vi "MCSPowerWriter.vi"(4 "ErrorIn":errorcluster, 5 "UDPResponse":string="\u0000\u0000PM\u001eš\n\u0000.¾\u0004\b\u0000\u0000\u00000\u0000\u0000\u00000\u0000\u0000\u00000\u0000\u0000\u00000\u0000\u0000\u00000«Î\u0004\b\u0000\u0000\u00000\u0000\u0000\u00000\u0000\u0000\u00000\u0000\u0000\u00000\u0000\u0000\u00000ÿÿÿÿ", 6 "MPDUnitID":T1=enum."MPD#04", 7 "PowerChannelMap":T2[](array[typedef])=[enum."WVOnline", enum."Unassigned", enum."Unassigned", enum."Unassigned", enum."Unassigned", enum."Unassigned", enum."WVOffline", enum."Unassigned", enum."Unassigned", enum."Unassigned", enum."Unassigned", enum."Unassigned"]) -> (0 "ErrorOut":errorcluster, 3 "ByteArray":u8[](array[numeric])=[64, 55, 34, 184, 91, 157, 14, 129, 0, 12, 0, 0, 0, 0, 0, 0, 1, 2, 3, 4, 5, 6, 0, 0, 80, 77, 30, 154, 10, 0, 46, 190, 4, 8, 0, 0, 0, 48, 0, 0, 0, 48, 0, 0, 0, 48, 0, 0, 0, 48, 0, 0, 0, 48, 171, 206, 4, 8, 0, 0, 0, 48, 0, 0, 0, 48, 0, 0, 0, 48, 0, 0, 0, 48, 0, 0, 0, 48, 255, 255, 255, 255, 13, 10])   [LabVIEW 2012]
uses:
  MCSPowerMap.ctl
  MPDUnitID.ctl
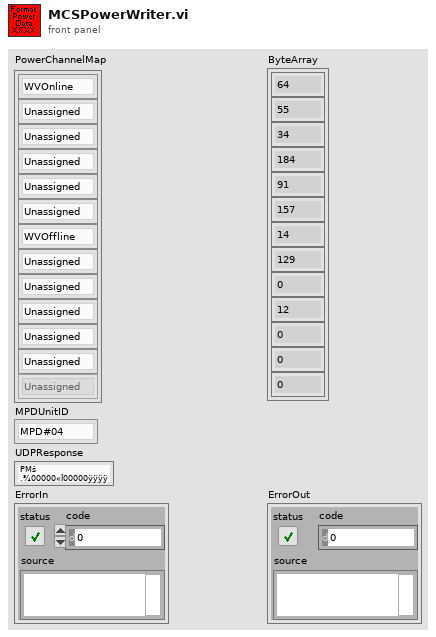
[diagram p1: front panel]
types:
  T1 = typedef "MPDUnitID.ctl" = enum8{"Unknown", "MPD#01", "MPD#02", "MPD#03", "MPD#04", "MPD#05"}
  T2 = typedef "MCSPowerMap.ctl" = enum8{"Unassigned", "Unknown", "WVOnline", "WVOffline", "O2Online", "O2Offline", "HSRL"}
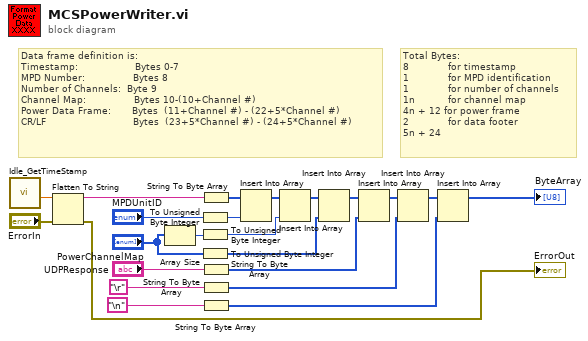
[diagram p0: block diagram]
diagram:
  # "Total Bytes:\n8             for timestamp\n1             for MPD identification\n1             for number of channels\n1n           for channel map\n4n + 12 for power frame\n2             for data footer\n5n + 24"
  # "Data frame definition is:\nTimestamp:                   Bytes 0-7\nMPD Number:                Bytes 8\nNumber of Channels:  Byte 9\nChannel Map:                Bytes 10-(10+Channel #)\nPower Data Frame:       Bytes  (11+Channel #) - (22+5*Channel #)\nCR/LF                             Bytes  (23+5*Channel #) - (24+5*Channel #)"
  n1 = call "Idle_GetTimeStamp.vi"() -> ("Fractional Hours"=w18:dbl)  [unwired: 11 in]
  n2 = Flatten To String(anything=w18, error in (no error)="ErrorIn") -> (data string=w19:string, error out=→"ErrorOut":errorcluster)  [unwired: 2 in, 1 out]
  n3 = Array Size(array="PowerChannelMap") -> (size(s)=w17:i32)
  n4 = To Unsigned Byte Integer(number="MPDUnitID") -> (unsigned 8bit integer=w3:u8)
  n5 = To Unsigned Byte Integer(number=w17) -> (unsigned 8bit integer=w16:u8)
  n6 = To Unsigned Byte Integer(number="PowerChannelMap") -> (unsigned 8bit integer=w15:u8[])
  n7 = String To Byte Array(string=w19) -> (unsigned byte array=w6:u8[])
  n8 = String To Byte Array(string="UDPResponse") -> (unsigned byte array=w13:u8[])
  n9 = String To Byte Array(string="\r") -> (unsigned byte array=w10:u8[])
  n10 = String To Byte Array(string="\n") -> (unsigned byte array=w20:u8[])
  n11 = Insert Into Array(array=w6, new element=w3) -> (w5:u8[])  [unwired: 1 in]
  n12 = Insert Into Array(array=w5, new element=w16) -> (w8:u8[])  [unwired: 1 in]
  n13 = Insert Into Array(array=w8, new element=w15) -> (w14:u8[])  [unwired: 1 in]
  n14 = Insert Into Array(array=w14, new element=w13) -> (w12:u8[])  [unwired: 1 in]
  n15 = Insert Into Array(array=w12, new element=w10) -> (w11:u8[])  [unwired: 1 in]
  n16 = Insert Into Array(array=w11, new element=w20) -> (→"ByteArray":u8[])  [unwired: 1 in]
